vi "HW Engine UI.vi"() -> ()   [LabVIEW 2025, in "HW Engine.lvlib" / "HW Engine.lvclass"]
doc: "Copyright 2017 National Instruments Corporation\n\nLicensed under the Apache License, Version 2.0 (the \"License\"); you may not use this file except in compliance with the License. You may obtain a copy of the License at http://www.apache.org/licenses/LICENSE-2.0\nUnless required by applicable law or agreed to in writing, software distributed under the License is distributed on an \"AS IS\" BASIS, WITHOUT WARRANTIES OR CONDITIONS OF ANY KIND, either express or implied. See the License for the specific language governing permissions and limitations under the License."
uses:
  HW Engine.lvclass
  Users/Public/Documents/Sandia National Labs/TSS Plugin/CEF.lvlibp/Node/UserEventRef.ctl
  Users/Public/Documents/Sandia National Labs/TSS Plugin/CEF.lvlibp/Node/mainQref.ctl
  Users/Public/Documents/Sandia National Labs/TSS Plugin/CEF.lvlibp/Node/NodeRef.ctl
  Users/Public/Documents/Sandia National Labs/TSS Plugin/CEF.lvlibp/Node/CEF_Node.lvclass
  Users/Public/Documents/Sandia National Labs/TSS Plugin/CEF.lvlibp
panel:
  out "Engine Status":i32(listbox)=-1
  in  "Segmented":T1(radio)=enum."Power Supply"
  in  "node ref":T2
  in  "Treeview":string(tree)="S3686"
  in  "main queue":T3
  in  "user event":T4
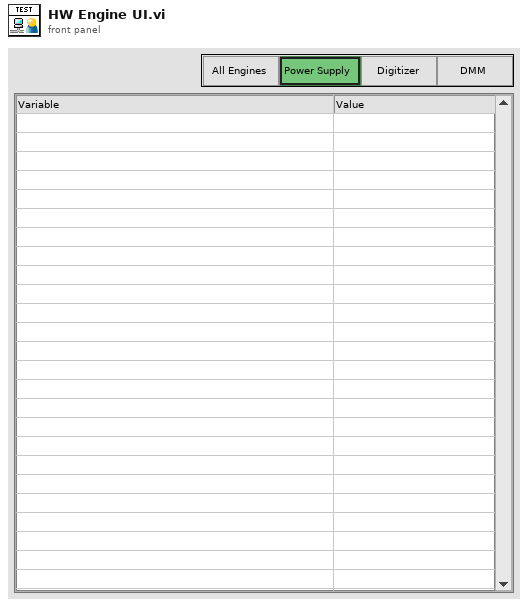
[diagram p1: front panel]
types:
  T1 = enum32{"All Engines", "Power Supply", "Digitizer", "DMM"}
  T2 = typedef "CEF.lvlibp/CEF_Node.lvclass/NodeRef.ctl" = refnum<data-value>
  T3 = typedef "CEF.lvlibp/CEF_Node.lvclass/mainQref.ctl" = refnum<queue>
  T4 = typedef "CEF.lvlibp/CEF_Node.lvclass/UserEventRef.ctl" = refnum<user-event>
  T5 = cluster{"Tag":string, "Text":string, "Parent Tag":string, "Value":string}[]
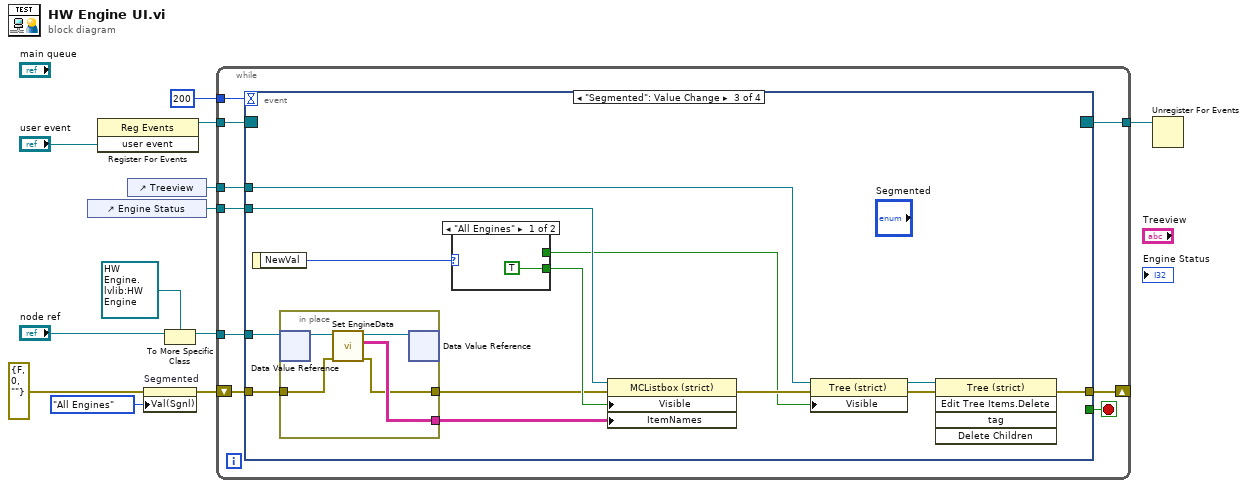
[diagram p0: block diagram]
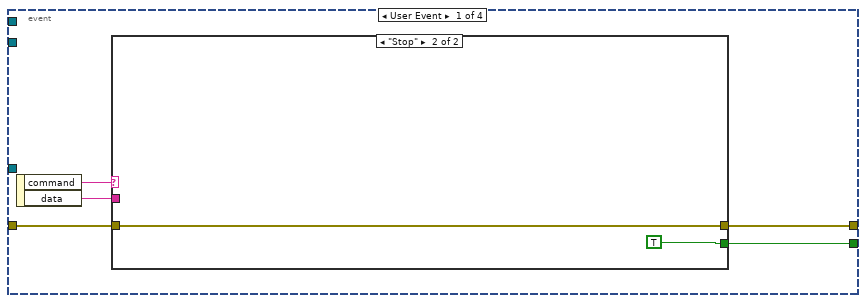
[diagram p2: hidden frame]
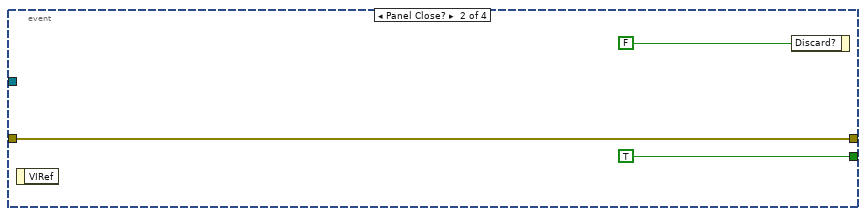
[diagram p4: hidden frame]
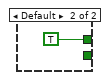
[diagram p5: hidden frame]
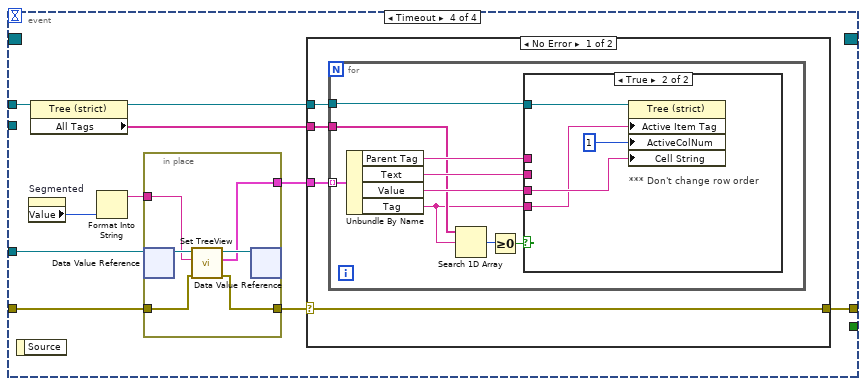
[diagram p6: hidden frame]
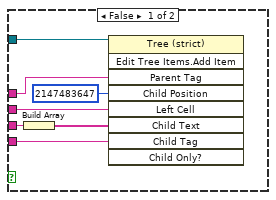
[diagram p7: hidden frame]
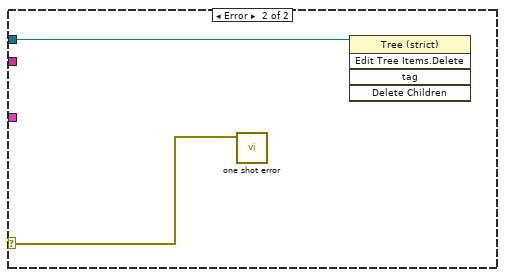
[diagram p8: hidden frame]
diagram:
  n1 = control-ref of="Engine Status"() -> (w4:refnum<vi>)
  n2 = register-events("user event") -> (reference out=w11:refnum<event-registration>)  [unwired: 2 in, 1 out]
  n3 = control-ref of="Treeview"() -> (w5:refnum<vi>)
  n4 = property on="Segmented" class="RadioBtnsControl (strict)"(error in=errorcluster {"status"=FALSE, "code"=0, "source"=""} ("error in (no error)"), "Val(Sgnl)"=T1."All Engines" ("Value (Signaling)")) -> (error out=w2:errorcluster)  [unwired: 1 in, 1 out]
  n5 = To More Specific Class(target class=refnum<data-value> refnum ("data value reference"), reference="node ref") -> (specific class reference=w6:refnum<data-value>)  [unwired: 1 in, 1 out]
  n6 = while {
    tunnel: w11 -> [w21]
    tunnel: [w20] -> w10
    shift-right: [w18] -> _
    shift-left: w2 -> [w17]
    tunnel: w6 -> [w16]
    tunnel: 200 -> [w15]
    tunnel: w5 -> [w14]
    tunnel: w4 -> [w13]
    stop <- w19 stop-if-true
    n7 = event shown="[2] \"Segmented\": Value Change" {
      selector: w21 -> [_ _ _ _]
      dyn-events: [_ _ _ _] -> w20
      timeout: w15 -> [_ _ _ _]
      tunnel: [w26 TRUE _ _] -> w19
      tunnel: [w24 w31 w43 w53] -> w18
      tunnel: w17 -> [w25 w31 w35 w56]
      tunnel: w16 -> [_ _ w37 w60]
      tunnel: w14 -> [_ _ w33 w59]
      tunnel: w13 -> [_ _ w42 _]
      event User Event {
        n8 = event-data() -> ("command"=w22:string, "data"=w23:string)  [unwired: 1 in]
        n9 = case shown="\"Stop\"" w22 {
          tunnel: w23 -> [_ _]
          tunnel: [_ TRUE] -> w26
          tunnel: w25 -> [w27 w28]
          tunnel: [w27 w28] -> w24
          frame Default {
          }
          frame "Stop" {
          }
        }
      }
      event Panel Close? {
        n10 = event-data() -> ()  [unwired: 1 in, 1 out]
        n11 = event-data("Discard?"=FALSE) -> ()  [unwired: 1 in, 1 out]
      }
      event "Segmented": Value Change {
        n12 = event-data() -> ("NewVal"=w40:T1)  [unwired: 1 in]
        n13 = in-place {
          in-place-border: [w49] -> w36
          in-place-border: w35 -> [w48]
          in-place-border: [w46] -> w34
          n14 = in-place-dvr #1(w37) -> (w50:refnum<class "HW Engine.lvclass">)  [unwired: 1 out]
          n15 = call "Set EngineData.vi"("error in (no error)"=w48, "HW Engine in"=w50) -> ("error out"=w46:errorcluster, "Engine DataSet"=w49:string[][], "HW Engine out"=w47:refnum<class "HW Engine.lvclass">)  [unwired: 7 in]
          n16 = in-place-dvr #1(w47) -> ()  [unwired: 2 out]
        }
        n17 = case shown="\"All Engines\"" w40 {
          tunnel: [_ TRUE ("Visible")] -> w39
          tunnel: [TRUE ("Visible") _] -> w38
          frame "All Engines" {
          }
          frame Default {
          }
        }
        n18 = property class="MCListbox (strict)"(reference=w42, error in=w34, "Visible"=w38, "ItemNames"=w36) -> (error out=w41:errorcluster)  [unwired: 1 out]
        n19 = property class="Tree (strict)"(reference=w33, error in=w41, "Visible"=w39) -> (reference out=w44:refnum<vi>, error out=w45:errorcluster)
        n20 = invoke class="Tree (strict)" method="Edit Tree Items.Delete"(reference=w44, error in=w45) -> (error out=w43:errorcluster)  [unwired: 3 in, 4 out]
      }
      event Timeout {
        n21 = event-data() -> ()  [unwired: 1 in, 1 out]
        n22 = property on="Segmented" class="RadioBtnsControl (strict)"() -> ("Value"=w62:T1)  [unwired: 2 in, 2 out]
        n23 = property class="Tree (strict)"(reference=w59) -> (reference out=w58:refnum<vi>, "All Tags"=w55:string[])  [unwired: 1 in, 1 out]
        n24 = Format Into String(w62) -> (resulting string=w61:string)  [unwired: 3 in, 1 out]
        n25 = in-place {
          in-place-border: w61 -> [w93]
          in-place-border: [w89] -> w57
          in-place-border: w56 -> [w91]
          in-place-border: [w90] -> w54
          n26 = in-place-dvr #2(w60) -> (w94:refnum<class "HW Engine.lvclass">)  [unwired: 1 out]
          n27 = call "Set TreeView.vi"("error in"=w91, "Engine"=w93, "HW Engine in"=w94) -> ("error out"=w90:errorcluster, "Tree DataSet"=w89:T5, "HW Engine out"=w92:refnum<class "HW Engine.lvclass">)  [unwired: 6 in]
          n28 = in-place-dvr #2(w92) -> ()  [unwired: 2 out]
        }
        n29 = case shown="No Error" w54 {
          selector: w54 -> [w63 w88]
          tunnel: w58 -> [w66 w87]
          tunnel: w57 -> [w65 _]
          tunnel: w55 -> [w64 _]
          tunnel: [w63 _] -> w53
          frame No Error {
            n30 = for {
              tunnel: w65 -> [w73] mode=indexing
              tunnel: w64 -> [w70]
              tunnel: w66 -> [w72]
              n31 = Unbundle By Name(w73) -> ("Parent Tag"=w75:string, "Text"=w74:string, "Value"=w71:string, "Tag"=w69:string)
              n32 = Search 1D Array(1D array=w70, element=w69) -> (index of element=w68:i32)  [unwired: 1 in]
              n33 = Greater Or Equal To 0?(x=w68) -> (x >= 0?=w67:bool)
              n34 = case shown="True" w67 {
                tunnel: w72 -> [w82 w86]
                tunnel: w69 -> [w80 w83]
                tunnel: w75 -> [w78 _]
                tunnel: w74 -> [w77 _]
                tunnel: w71 -> [w76 w85]
                frame False {
                  n35 = Build Array(w76) -> (w81:string[])
                  n36 = invoke class="Tree (strict)" method="Edit Tree Items.Add Item"(reference=w82, "Parent Tag"=w78, "Child Position"=2147483647, "Left Cell"=w77, "Child Text"=w81, "Child Tag"=w80) -> ()  [unwired: 3 in, 9 out]
                }
                frame True {
                  # "*** Don't change row order"
                  n37 = property class="Tree (strict)"(reference=w86, "Active Item Tag"=w83, "ActiveColNum"=1 ("Active Cell:Active Column Number"), "Cell String"=w85) -> ()  [unwired: 1 in, 2 out]
                }
              }
            }
          }
          frame Error {
            n38 = call "one shot error.vi"("error in"=w88) -> ()  [unwired: 11 in]
            n39 = invoke class="Tree (strict)" method="Edit Tree Items.Delete"(reference=w87) -> ()  [unwired: 4 in, 5 out]
          }
        }
      }
    }
  }
  n40 = Unregister For Events(event registration refnum=w10) -> ()  [unwired: 1 in, 1 out]
